vi "RichToFlatnise_OpenSessionInputs.vi"(5 "OutputClusterType":T1, 11 "InputCluster":T2) -> (3 "OutputCluster":T1)   [LabVIEW 2021, in "basic_switch_executive_driver_client.lvlib"]
uses:
  basic_switch_executive_driver_client.lvlib
  nise_OpenSessionInputs.ctl
  <vilib>/Plug-In SDKs/Clients/Session Management V1/Session Reservation/Initialize and Close Session Behavior.ctl
  nise_OpenSessionInputs_Flat.ctl
  <vilib>/Plug-In SDKs/Clients/Session Management V1/Session Reservation/Session Reservation.lvclass
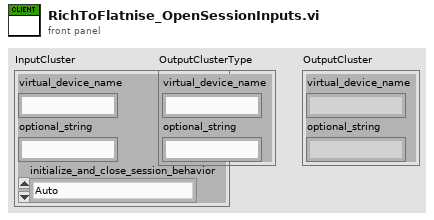
[diagram p1: front panel]
types:
  T1 = typedef "basic_switch_executive_driver_client.lvlib/nise_OpenSessionInputs_Flat.ctl" = cluster{"virtual_device_name":string, "optional_string":string}
  T2 = typedef "basic_switch_executive_driver_client.lvlib/nise_OpenSessionInputs.ctl" = cluster{"virtual_device_name":string, "optional_string":string, "initialize_and_close_session_behavior":T3}
  T3 = typedef "NI Session Management V1 Client.lvlib/Session Reservation.lvclass/Initialize and Close Session Behavior.ctl" = enum16{"Auto", "Initialize and Close", "Attach and Detach", "Initialize and Detach", "Attach and Close"}
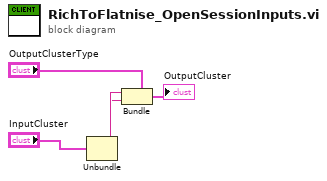
[diagram p0: block diagram]
diagram:
  n1 = Unbundle "Unbundle"("InputCluster") -> ("virtual_device_name"=w2:string, "optional_string"=w1:string)  [unwired: 1 out]
  n2 = Bundle "Bundle"(cluster="OutputClusterType", "virtual_device_name"=w2, "optional_string"=w1) -> (→"OutputCluster":T1)
